vi "Analog Input - N Channels - N Samples.vi"() -> ()   [LabVIEW 2019]
uses:
  <vilib>/myRIO/Common/Instrument Driver Framework/ELVIS III v1.0/AI Block/vis/ELVIS III v1.0 AI Block Read.vi
  <vilib>/myRIO/Common/Instrument Driver Framework/ELVIS III v1.0/AI Block/vis/ELVIS III v1.0 Close AI Block.vi
  <vilib>/myRIO/Common/Instrument Driver Framework/myRIO v1.0/UART/vis/myRIO v1.0 Close UART.vi
  <vilib>/myRIO/Common/Instrument Driver Framework/Utilities/vis/Sample Rate To Ticks.vi
  <vilib>/myRIO/Common/Instrument Driver Framework/ELVIS III v1.0/AI Block/vis/ELVIS III v1.0 Unreserve AI Block.vi
  <vilib>/myRIO/Common/Instrument Driver Framework/ELVIS III v1.0/AI Block/vis/ELVIS III v1.0 Build MUX Configuration AI Block.vi
  <vilib>/Utility/error.llb/Error Cluster From Error Code.vi
  <vilib>/myRIO/Common/Instrument Driver Framework/myRIO v1.0/Resource Manager/vis/myRIO v1.0 Block Write Configuration.vi
  <vilib>/myRIO/Common/Instrument Driver Framework/ELVIS III v1.0/AI Block/vis/ELVIS III v1.0 AI Block Read Bank A.vi
  <vilib>/myRIO/Common/Instrument Driver Framework/ELVIS III v1.0/AI Block/vis/ELVIS III v1.0 AI Block Read Bank B.vi
  <vilib>/myRIO/Common/Instrument Driver Framework/ELVIS III v1.0/Resource Manager/vis/ELVIS III v1.0 Unreserve Channel List.vi
  <vilib>/myRIO/Common/Instrument Driver Framework/myRIO v1.0/myRIO v1.0 Close.vi
  <vilib>/myRIO/Common/Instrument Driver Framework/Utilities/vis/FPGA Ref Manager.vi
  <vilib>/myRIO/Common/Instrument Driver Framework/ELVIS III v1.0/ELVIS III v1.0 Reset FPGA.vi
  <vilib>/myRIO/Common/Instrument Driver Framework/myRIO v1.0/IRQ/vis/myRIO v1.0 IRQ Info FGV.vi
  <vilib>/myRIO/Common/Instrument Driver Framework/myRIO v1.0/IRQ/vis/myRIO v1.0 Timer IRQ Info FGV.vi
  <vilib>/myRIO/Common/Instrument Driver Framework/myRIO v1.0/IRQ/vis/myRIO v1.0 ISR Agent.vi
  <vilib>/myRIO/Instrument Drivers/Utilities/vis/Reset Index.vi
  <vilib>/myRIO/Common/Instrument Driver Framework/myRIO v1.0/Resource Manager/vis/myRIO v1.0 Block Write Resource Manager.vi
  <vilib>/myRIO/Instrument Drivers/Utilities/Utilities.lvlib
  <vilib>/myRIO/Instrument Drivers/Onboard IO/AI Block/AI Block.lvlib
panel:
  in  "Acquire Data":bool
  in  "Stop":bool
  out "Analog Data":dbl[][](graph)
  # "ELVIS III Control IO"
  # "模拟输入N通道"
  # "Overview: Acquires N sample voltage values from Bank A, Channel 0 and 1 (A/AI0 and A/AI1).\nInstructions:\n1. Connect A/AI0 and A/AI1 to valid signals.\n2. Run the VI.\n3. Click Acquire Data to trigger an acquisition."
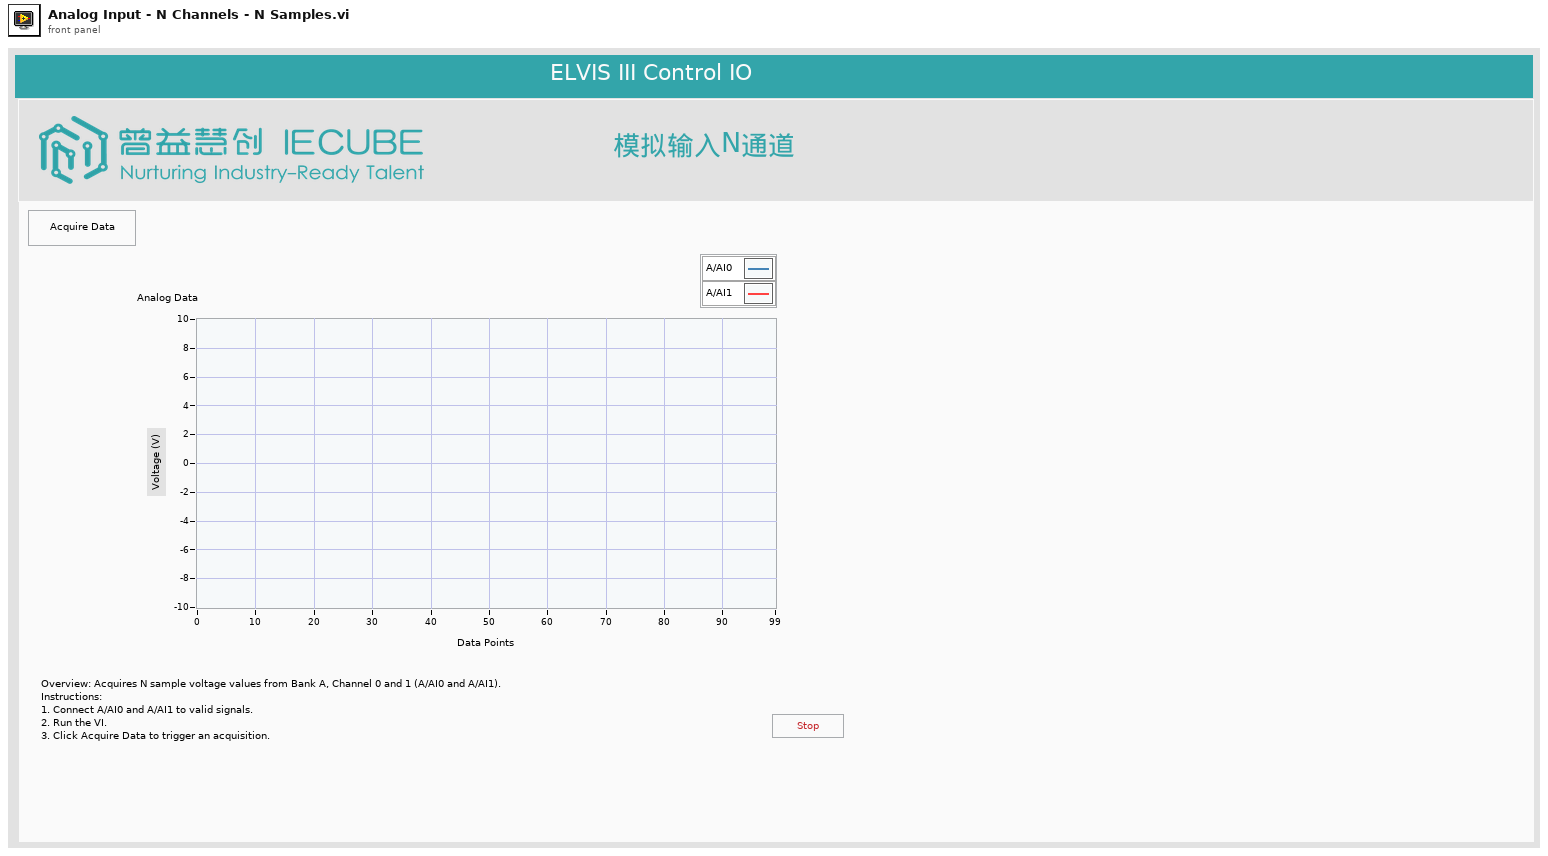
[diagram p1: front panel]
types:
  T1 = typedef "AI Block.lvlib/AI Block Reference.ctl" = cluster{"myRIO Reference":T2, "AI (N Samples) Channels List":T6, "AI (N Samples) Scaling Constants List":T8[]}
  T2 = typedef "myRIO Generic Hardware Reference.ctl" = cluster{"myRIO Model":T3, "myRIO Hardware Reference":T4}
  T3 = typedef "Hardware Version Enum.ctl" = enum16{"Unknown", "myRIO-1900", "myRIO-1950", "roboRIO", "NI ELVIS RIO CM", "ELVIS III"}
  T4 = typedef "myRIO v1.0 Reference.ctl" = cluster{"Generic FPGA Reference":T5, "Allow multiple opens":bool}
  T5 = typedef "Generic FPGA Reference.ctl" = refnum<k20>
  T6 = typedef "AI Block Channels List.ctl" = T7[]
  T7 = typedef "AI Block Channels Enum.ctl" = enum16{"Not Connected", "A/AI0 (N Samples)", "A/AI1 (N Samples)", "A/AI2 (N Samples)", "A/AI3 (N Samples)", "A/AI4 (N Samples)", "A/AI5 (N Samples)", "A/AI6 (N Samples)", "A/AI7 (N Samples)", "A/AI0 (DIFF N Samples)", "A/AI1 (DIFF N Samples)", "A/AI2 (DIFF N Samples)", "A/AI3 (DIFF N Samples)", "B/AI0 (N Samples)", "B/AI1 (N Samples)", "B/AI2 (N Samples)", "B/AI3 (N Samples)", "B/AI4 (N Samples)", "B/AI5 (N Samples)", "B/AI6 (N Samples)", "B/AI7 (N Samples)", "B/AI0 (DIFF N Samples)", "B/AI1 (DIFF N Samples)", "B/AI2 (DIFF N Samples)", "B/AI3 (DIFF N Samples)"}
  T8 = typedef "Analog Scaling Constants.ctl" = cluster{"LSB Weight (Volts)":dbl, "Offset (Volts)":dbl, "Signed?":bool}
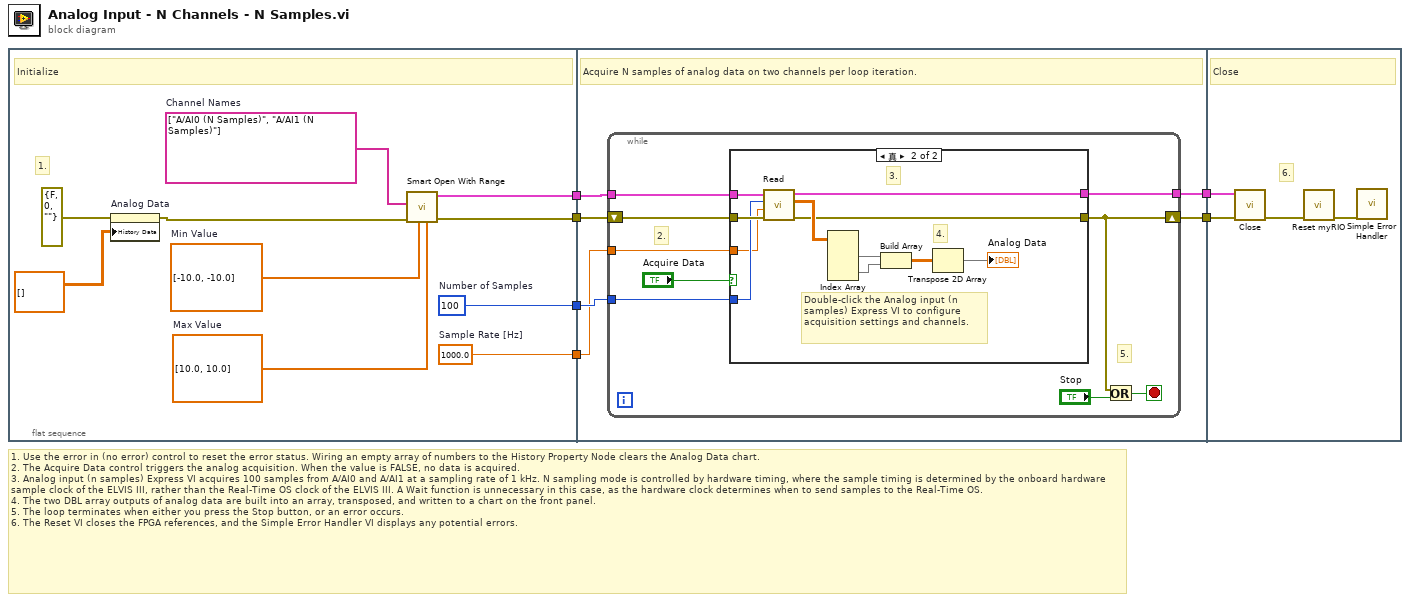
[diagram p0: block diagram]
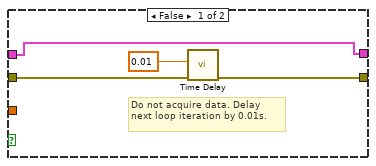
[diagram p2: hidden frame]
diagram:
  # "1. Use the error in (no error) control to reset the error status. Wiring an empty array of numbers to the History Property Node clears the Analog Data chart. \n2. The Acquire Data control triggers the analog acquisition. When the value is FALSE, no data is acquired.\n3. Analog input (n samples) Express VI acquires 100 samples from A/AI0 and A/AI1 at a sampling rate of 1 kHz. N sampling mode is controlled by hardware timing, where the sample timing is determined by the onboard hardware sample clock of the ELVIS III, rather than the Real-Time OS clock of the ELVIS III. A Wait function is unnecessary in this case, as the hardware clock determines when to send samples to the Real-Time OS.\n4. The two DBL array outputs of analog data are built into an array, transposed, and written to a chart on the front panel.\n5. The loop terminates when either you press the Stop button, or an error occurs.\n6. The Reset VI closes the FPGA references, and the Simple Error Handler VI displays any potential errors."
  n1 = flat-sequence {
    tunnel: [w10] -> w5
    tunnel: [w9] -> w4
    tunnel: [w8] -> w3
    tunnel: [w7] -> w2
    tunnel: [w22] -> w6
    tunnel: w5 -> [w21]
    tunnel: w4 -> [w20]
    tunnel: w3 -> [w19]
    tunnel: w2 -> [w18]
    tunnel: [w17] -> w1
    tunnel: w6 -> [w49]
    tunnel: w1 -> [w47]
    frame #0 {
      w7 = 1000.0  # Sample Rate [Hz]
      w8 = u32 100  # Number of Samples
      w12 = dbl[] [10.0, 10.0]  # Max Value
      w13 = dbl[] [-10.0, -10.0]  # Min Value
      w14 = tag[] ["A/AI0 (N Samples)", "A/AI1 (N Samples)"]  # Channel Names
      # "1."
      # "Initialize"
      n2 = property on="Analog Data" class="WFChart (严格)"(error in=errorcluster {"status"=FALSE, "code"=0, "source"=""} ("error in (no error)"), "History Data"=dbl[][] []) -> (error out=w11:errorcluster)  [unwired: 1 in, 1 out]
      n3 = call <vilib>:"Smart Open With Range.vi"("Max Value"=w12, "Min Value"=w13, "error in (no error)"=w11, "Channel Names"=w14) -> ("error out"=w10:errorcluster, "AI (N Samples) Ref Out"=w9:T1)  [unwired: 6 in]
    }
    frame #1 {
      # "Acquire N samples of analog data on two channels per loop iteration."
      n4 = while {
        shift-right: [w29] -> w22
        shift-left: w21 -> [w30]
        tunnel: w20 -> [w23]
        tunnel: w19 -> [w26]
        tunnel: w18 -> [w25]
        tunnel: [w24] -> w17
        stop <- w31 stop-if-true
        # "5."
        # "2."
        n5 = case shown="真" "Acquire Data" {
          tunnel: w30 -> [w34 w45]
          tunnel: [w33 w42] -> w29
          tunnel: w26 -> [_ w44]
          tunnel: w25 -> [_ w43]
          tunnel: [w32 w37] -> w24
          tunnel: w23 -> [w32 w36]
          frame False {
            # "Do not acquire data. Delay next loop iteration by 0.01s."
            n6 = call "Time Delay"("error in (no error)"=w34, "Delay Time (s)"=0.01) -> ("error out"=w33:errorcluster)  [unwired: 9 in]
          }
          frame True {
            # "4."
            # "3."
            # "Double-click the Analog input (n samples) Express VI to configure acquisition settings and channels."
            n7 = call <vilib>:"Read.vi"("error in (no error)"=w45, "Sample Rate [Hz]"=w43, "Number of Samples"=w44, "AI (N Samples) Ref In"=w36) -> ("error out"=w42:errorcluster, "Values"=w46:dbl[][], "AI (N Samples) Ref Out"=w37:T1)  [unwired: 5 in]
            n8 = Index Array(array=w46) -> (element #1=w41:dbl[], element #2=w40:dbl[])  [unwired: 4 in]
            n9 = Build Array(w41, w40) -> (w39:dbl[][])
            n10 = Transpose 2D Array(2D array=w39) -> (transposed array=→"Analog Data":dbl[][])
          }
        }
        n11 = Or(x=w29, y="Stop") -> (x .or. y?=w31:bool)
      }
    }
    frame #2 {
      # "6."
      # "Close"
      n12 = call <vilib>:"Close.vi"("error in (no error)"=w49, "AI (N Samples) Ref In"=w47) -> ("error out"=w48:errorcluster)  [unwired: 9 in]
      n13 = call <vilib>:"Reset myRIO.vi"("error in (no error)"=w48) -> ("error out"=w50:errorcluster)  [unwired: 10 in]
      n14 = call <vilib>:"Simple Error Handler.vi"("error in (no error)"=w50) -> ()  [unwired: 4 in, 5 out]
    }
  }
